vi "Hello World.vi"() -> ()   [LabVIEW 2020]
panel:
  out "Var":string
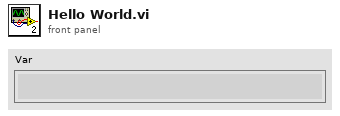
[diagram p1: front panel]
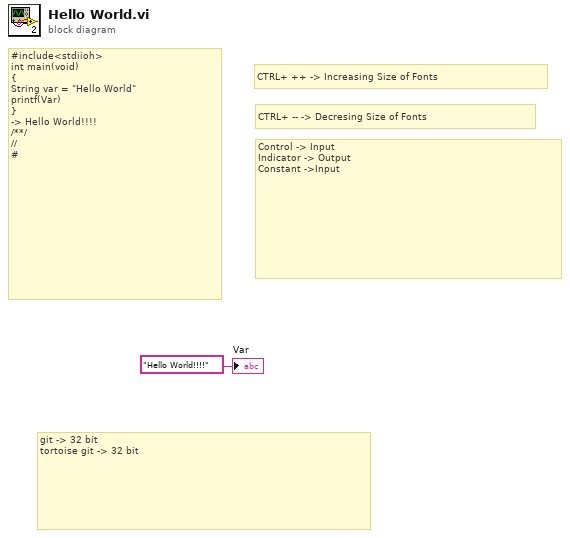
[diagram p0: block diagram]
diagram:
  # "git -> 32 bit\ntortoise git -> 32 bit"
  # "Control -> Input\nIndicator -> Output\nConstant ->Input"
  # "CTRL+ -- -> Decresing Size of Fonts"
  # "CTRL+ ++ -> Increasing Size of Fonts"
  # "#include<stdiioh>\nint main(void)\n{\nString var = \"Hello World\"\nprintf(Var)\n}\n-> Hello World!!!!\n/**/\n//\n#"
  "Var" <- "Hello World!!!!"
